vi "ProgressUI.vi"(6 "Message":string, 8 "error in (no error)":errorcluster, 9 "Time Remaining":dbl, 10 "Progress Bar":dbl, 11 "Settings":refnum<class "Progress Bar Settings.lvclass">) -> (0 "error out":errorcluster, 2 "Aborted":bool)   [LabVIEW 2016, in "Progress Bar.lvclass"]
doc: "The default UI that is shown to the user. This VI will pop up when a loop is entered\n\nCopyright: MGI\nAuthored by: Derek Trepanier"
uses:
  <userlib>/_MGI/User Interface/Progress Bar/Progress Bar.lvclass
  <userlib>/_MGI/User Interface/Progress Bar/Progress Bar Settings/Progress Bar Settings.lvclass
panel:
  in  "Abort":bool
  out "Time Remaining":dbl
  out "Progress Bar":dbl(slide) scale=0.0..1.0
  out "Message":string
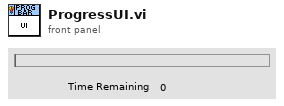
[diagram p1: front panel]
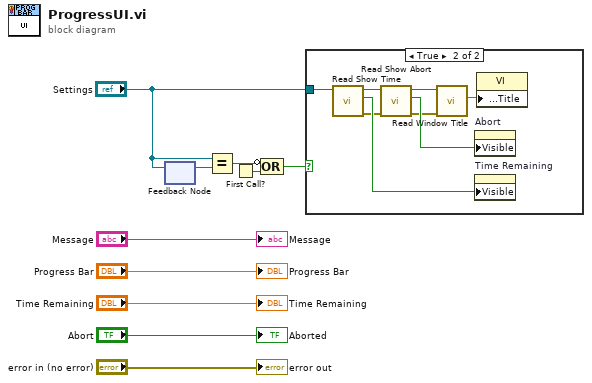
[diagram p0: block diagram]
diagram:
  n1 = feedback-in #1("Settings") -> ()
  n2 = feedback #1() -> (w3:refnum<class "Progress Bar Settings.lvclass">)  [unwired: 1 in]
  n3 = Equal?(x="Settings", y=w3) -> (x = y?=w2:bool)
  n4 = First Call?() -> (First Call?: T/F=w5:bool)
  n5 = Compound Arithmetic op=OR(invert w2, w5) -> (w1:bool)
  n6 = case shown="True" w1 {
    tunnel: "Settings" -> [_ w18]
    frame False {
    }
    frame True {
      n7 = call-dynamic "Read Show Time.vi"("MGI_Progress Bar Options in"=w18) -> ("error out"=w13:errorcluster, "Show Time"=w15:bool, "MGI_Progress Bar Options out"=w14:refnum<class "Progress Bar Settings.lvclass">)  [unwired: 8 in]
      n8 = call-dynamic "Read Show Abort.vi"("error in (no error)"=w13, "MGI_Progress Bar Options In"=w14) -> ("error out"=w11:errorcluster, "Show Abort"=w17:bool, "MGI_Progress Bar Options Out"=w12:refnum<class "Progress Bar Settings.lvclass">)  [unwired: 7 in]
      n9 = call-dynamic "Read Window Title.vi"("error in (no error)"=w11, "MGI_Progress Bar Options In"=w12) -> ("Window Title"=w16:string)  [unwired: 7 in, 2 out]
      n10 = property on="Abort" class="Bool"("Visible"=w17) -> ()  [unwired: 2 in, 2 out]
      n11 = property on="Time Remaining" class="DigNum (strict)"("Visible"=w15) -> ()  [unwired: 2 in, 2 out]
      n12 = property class="VI"("Front Panel.Title"=w16) -> ()  [unwired: 2 in, 2 out]
    }
  }
  "error out" <- "error in (no error)"
  "Message" <- "Message"
  "Progress Bar" <- "Progress Bar"
  "Time Remaining" <- "Time Remaining"
  "Aborted" <- "Abort"
